vi "Start Async.vi"(8 "error in (no error)":errorcluster, 11 "gRPC Server in":refnum<class "ctet_mux.lvclass">) -> (0 "error out":errorcluster, 3 "gRPC Server out":refnum<class "ctet_mux.lvclass">)   [LabVIEW 2019, in "ctet_mux.lvlib" / "ctet_mux.lvclass"]
uses:
  ctet_mux.lvclass
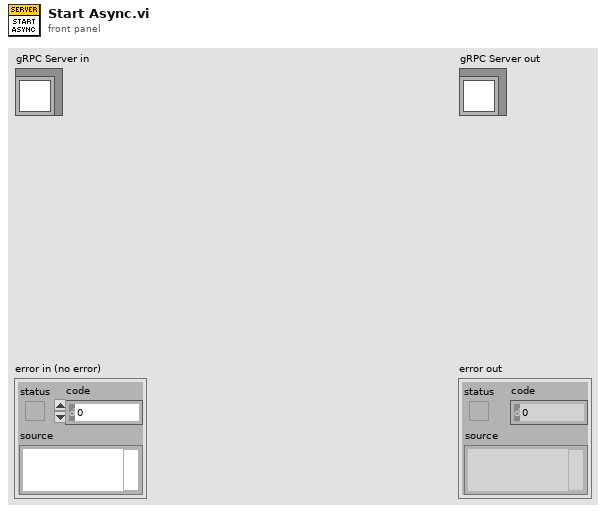
[diagram p1: front panel]
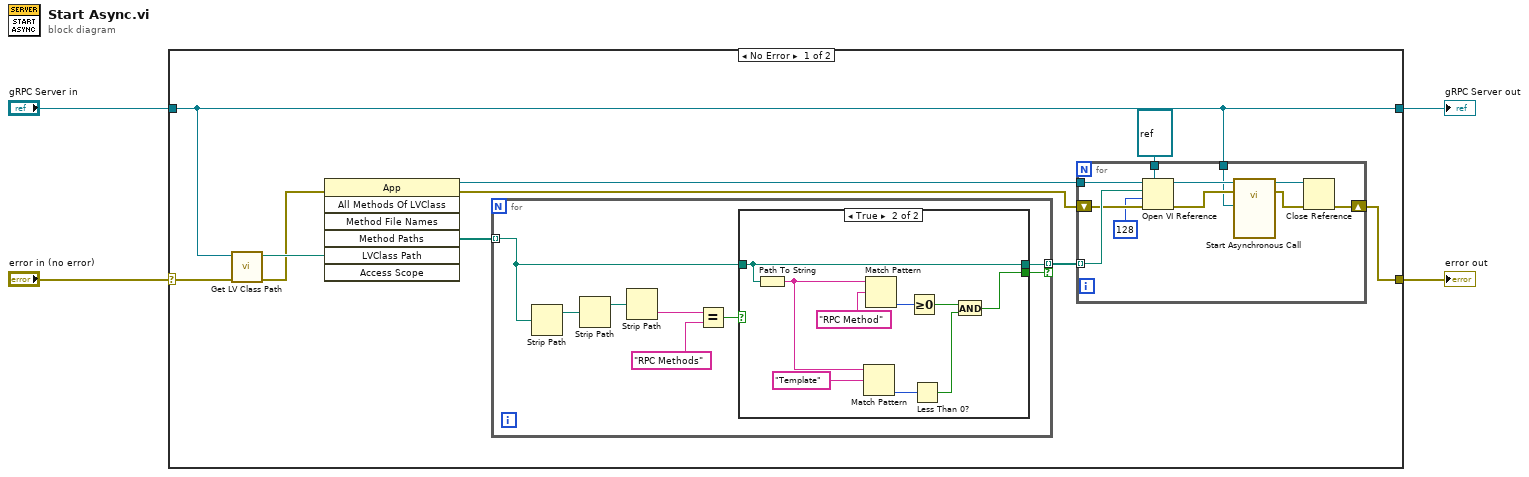
[diagram p0: block diagram]
diagram:
  n1 = case shown="No Error" "error in (no error)" {
    selector: "error in (no error)" -> [w10 w45]
    tunnel: [w7 w45] -> w3
    tunnel: [w11 w44] -> w1
    tunnel: "gRPC Server in" -> [w11 w44]
    frame No Error {
      n2 = call <vilib>:"Get LV Class Path.vi"("error in (no error)"=w10, "object"=w11) -> ("error out"=w8:errorcluster, "class path"=w14:path)  [unwired: 8 in]
      n3 = invoke class="App" method="All Methods Of LVClass"(error in=w8, "LVClass Path"=w14) -> (reference out=w12:refnum<vi>, error out=w9:errorcluster, "Method Paths"=w6:path[])  [unwired: 5 in, 4 out]
      n4 = for {
        tunnel: w6 -> [w20] mode=indexing
        tunnel: [w15] -> w5 mode=indexing if=w22
        n5 = Strip Path(path=w20) -> (stripped path=w21:path)  [unwired: 1 out]
        n6 = Strip Path(path=w21) -> (stripped path=w19:path)  [unwired: 1 out]
        n7 = Strip Path(path=w19) -> (name=w17:string)  [unwired: 1 out]
        n8 = Equal?(x=w17, y="RPC Methods" ("name")) -> (x = y?=w16:bool)
        n9 = case shown="True" w16 {
          tunnel: [_ w24] -> w22
          tunnel: w20 -> [w23 w30]
          tunnel: [w23 w30] -> w15
          frame False {
          }
          frame True {
            n10 = Path To String(path=w30) -> (string=w29:string)
            n11 = Match Pattern(string=w29, regular expression="Template") -> (offset past match=w27:i32)  [unwired: 1 in, 3 out]
            n12 = Match Pattern(string=w29, regular expression="RPC Method") -> (offset past match=w31:i32)  [unwired: 1 in, 3 out]
            n13 = Greater Or Equal To 0?(x=w31) -> (x >= 0?=w26:bool)
            n14 = Less Than 0?(x=w27) -> (x < 0?=w25:bool)
            n15 = And(x=w26, y=w25) -> (x .and. y?=w24:bool)
          }
        }
      }
      n16 = for {
        tunnel: w5 -> [w43] mode=indexing
        tunnel: refnum<vi> refnum ("type specifier VI Refnum (for type only)") -> [w42]
        tunnel: w12 -> [w39]
        tunnel: w11 -> [w36]
        shift-right: [w34] -> w7
        shift-left: w9 -> [w35]
        n17 = Open VI Reference(type specifier VI Refnum (for type only)=w42, application reference (local)=w39, vi path=w43, options=128 ("call and forget"), error in (no error)=w35) -> (vi reference=w41:refnum<vi>, error out=w38:errorcluster)  [unwired: 1 in]
        n18 = call-by-ref "Start Asynchronous Call"(reference=w41, error in=w38, "OOP Server in"=w36) -> (reference out=w40:refnum<vi>, error out=w37:errorcluster)  [unwired: 9 in, 2 out]
        n19 = Close Reference(reference=w40, error in (no error)=w37) -> (error out=w34:errorcluster)
      }
    }
    frame Error {
    }
  }
  "error out" <- w3
  "gRPC Server out" <- w1
